vi "Trigger Gate.vi"(8 "Offset (0)":i32, 9 "Threshold":dbl format="%0.2f", 11 "Waveform":dbl[](array[numeric])) -> (0 "Satisfied":bool, 1 "Stop":u32, 3 "Start":u32)   [LabVIEW 2013]
uses:
  <vilib>/express/express signal manip/TriggerBlock.llb/triggerSense.ctl
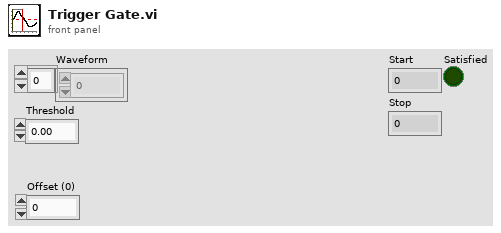
[diagram p1: front panel]
types:
  T1 = typedef "triggerSense.ctl" = enum32{"Rising", "Rising or Falling", "Falling"}
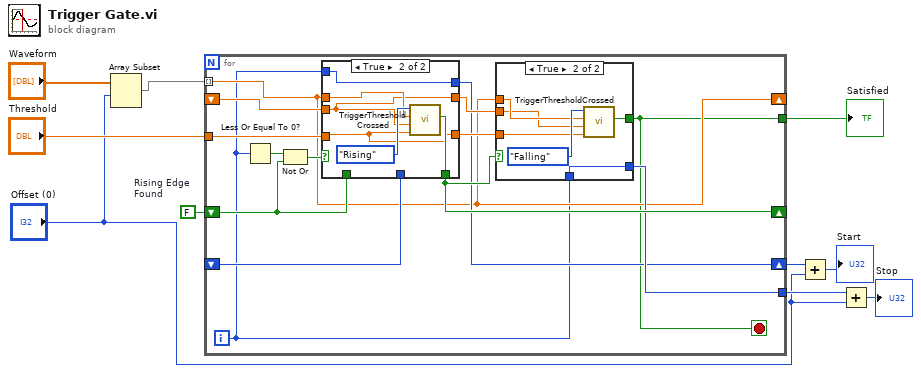
[diagram p0: block diagram]
diagram:
  w9 = FALSE  # Rising Edge Found
  n1 = Array Subset(array="Waveform", index="Offset (0)") -> (w8:dbl[])  [unwired: 1 in]
  n2 = for {
    tunnel: w8 -> [w13] mode=indexing
    shift-right: [w13] -> _
    shift-left: _ -> [w24]
    tunnel: "Threshold" -> [w23]
    shift-right: [w19] -> _
    shift-left: w9 -> [w20]
    tunnel: [w16] -> w4
    shift-right: [w15] -> w5
    shift-left: _ -> [w14]
    tunnel: [w11] -> w1
    i -> [w12]
    stop <- w11 stop-if-true
    n3 = Less Or Equal To 0?(x=w12) -> (x <= 0?=w22:bool)
    n4 = Not Or(1:w20, 2:w22) -> (0:w21:bool)
    n5 = case shown="True" w21 {
      tunnel: w13 -> [_ w38]
      tunnel: w24 -> [w35 w37]
      tunnel: w23 -> [w34 w40]
      tunnel: [w36 w41] -> w19
      tunnel: w20 -> [w36 _]
      tunnel: [w35 w37] -> w18
      tunnel: [w34 w40] -> w17
      tunnel: [w33 w39] -> w15
      tunnel: w14 -> [w33 _]
      tunnel: w12 -> [_ w39]
      frame False {
      }
      frame True {
        n6 = call "TriggerThresholdCrossed.vi"("Threshold"=w40, "Last"=w37, "Current"=w38, "Sense"=triggerSense."Rising") -> ("Satisfied"=w41:bool)  [unwired: 7 in]
      }
    }
    n7 = case shown="True" w19 {
      selector: w19 -> [w26 _]
      tunnel: w13 -> [_ w28]
      tunnel: [w25 w29] -> w16
      tunnel: w18 -> [_ w27]
      tunnel: w17 -> [_ w31]
      tunnel: [w26 w30] -> w11
      tunnel: w12 -> [w25 w29]
      frame False {
      }
      frame True {
        n8 = call "TriggerThresholdCrossed.vi"("Threshold"=w31, "Last"=w27, "Current"=w28, "Sense"=triggerSense."Falling") -> ("Satisfied"=w30:bool)  [unwired: 7 in]
      }
    }
  }
  "Satisfied" <- w1
  n9 = Add(x=w5, y="Offset (0)") -> (x+y=→"Start":i32)
  n10 = Add(x=w4, y="Offset (0)") -> (x+y=→"Stop":i32)
